vi "CodigoLabView 3.2.vi"() -> (11 "Releb 2":bool)   [LabVIEW 2025]
uses:
  <vilib>/Utility/NIReport.llb/Report Type.ctl
  <vilib>/Instr/_visa.llb/VISA Configure Serial Port (Instr).vi
  <vilib>/addons/_office/excel.llb/Excel Easy Table (str).vi
  <vilib>/Utility/NIReport.llb/NI_report.lvclass
  <vilib>/addons/_office/NI_ReportGenerationToolkit.lvlib
  <vilib>/Utility/NIReport.llb/NI_ReportGenerationCore.lvlib
  <vilib>/Utility/NIReport.llb/Excel/NI_Excel.lvclass
panel:
  out "Presionado":bool
  in  "RUTA DE REGISTRO":path
  out "Reloj Pot 4":dbl(knob) scale=0.0..100.0
  out "Reloj Pot 3":dbl(knob) scale=0.0..100.0
  out "Reloj Pot 2":dbl(knob) scale=0.0..100.0
  out "R ON 4":bool
  out "R ON 3":bool
  out "R ON 2":bool
  out "?":string
  out "R ON 1":bool
  out "TENSIÓN DE LÍNEA":dbl(knob) scale=100.0..300.0
  out "Reloj Pot 1":dbl(knob) scale=0.0..100.0
  in  "?":bool
  out "Releb 4":bool
  out "Relea 4":bool
  out "Rele 4":bool
  out "TOMACORRIENTE 4":bool
  out "Estado 4":string
  in  "Relé N°4":bool
  out "Potencia 4":string
  out "Releb 3":bool
  out "Relea 3":bool
  out "Rele 3":bool
  out "TOMACORRIENTE 3":bool
  out "Estado 3":string
  out "Potencia 3":string
  in  "Relé N°3":bool
  out "Relea 2":bool
  out "Rele 2":bool
  out "TOMACORRIENTE 2":bool
  out "Estado 2":string
  out "Potencia 2":string
  in  "Relé N°2":bool
  out "Releb 1":bool
  out "Relea 1":bool
  out "Rele 1":bool
  out "TOMACORRIENTE 1":bool
  out "Estado 1":string
  out "Potencia 1":string
  in  "Relé N°1":bool
  in  "PUERTO DE COMUNICACIÓN":refnum<visa-resource-name>
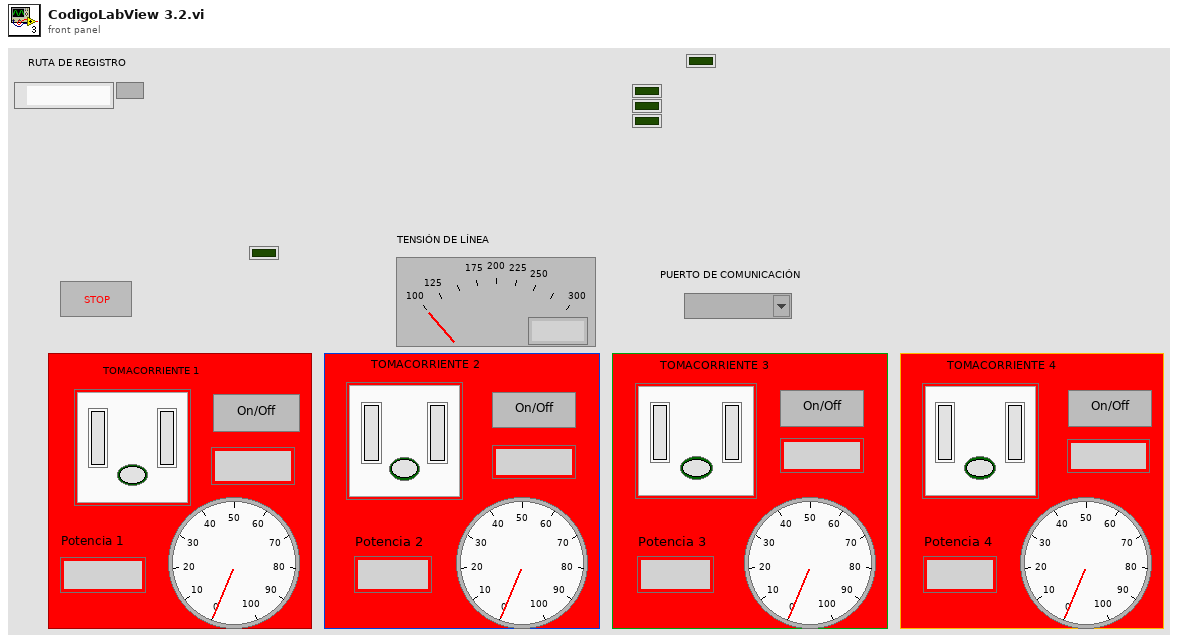
[diagram p1: front panel]
types:
  T1 = typedef "NI_ReportGenerationCore.lvlib/Report Type.ctl" = enum16{"HTML", "Word", "Excel"}
  T2 = cluster{"W1":string, "W2":string, "W3":string, "W4":string, "V":string}
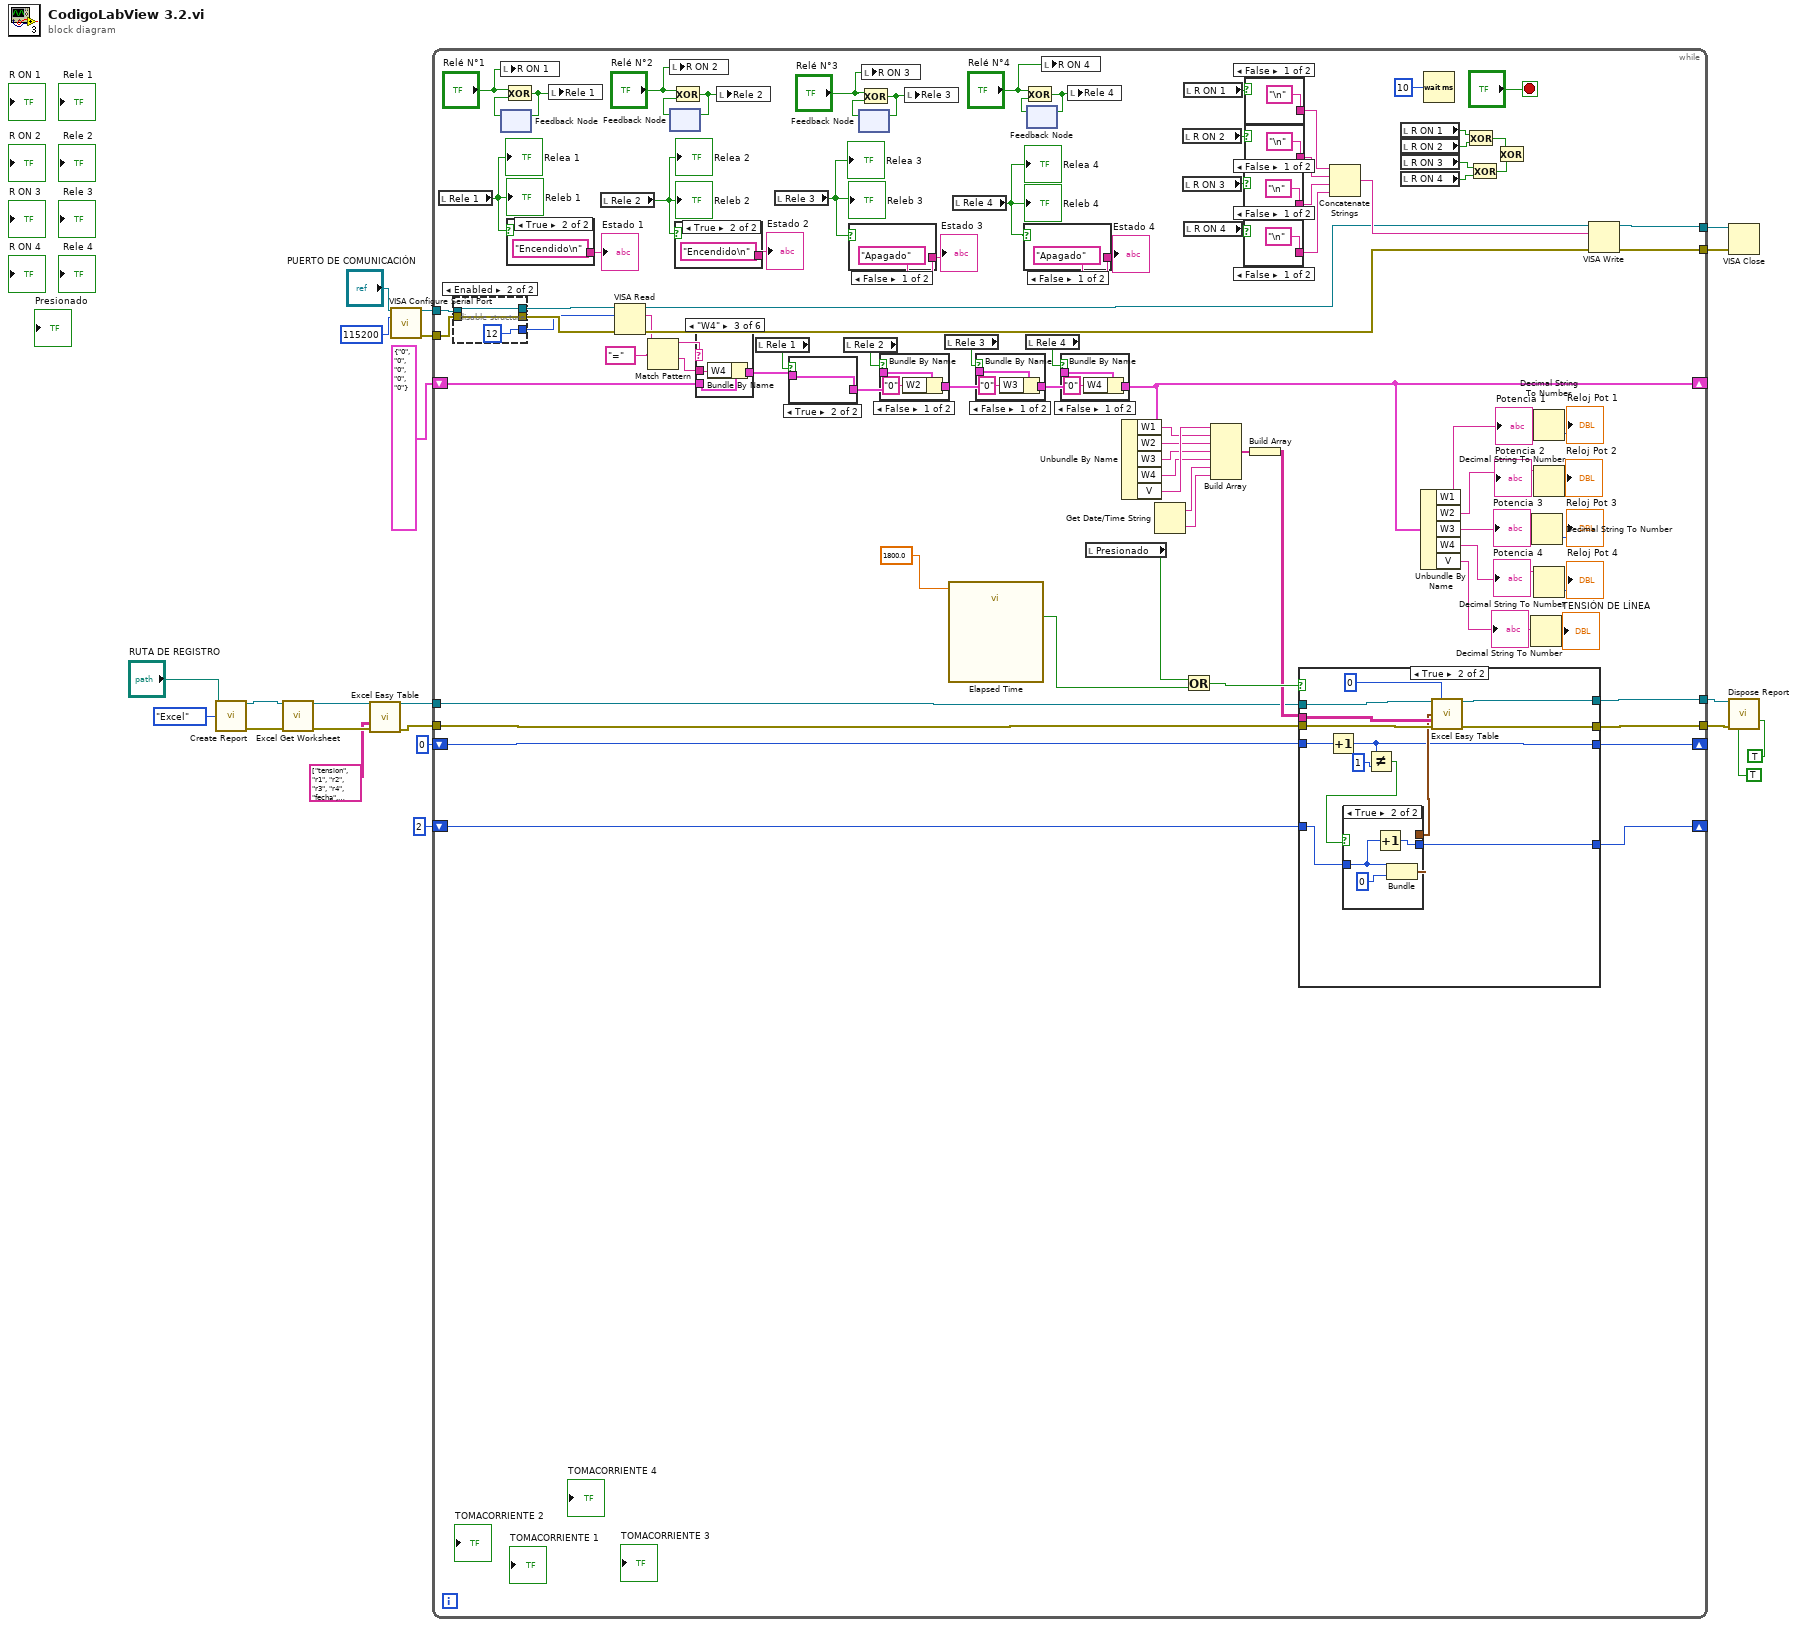
[diagram p0: block diagram]
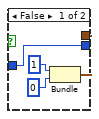
[diagram p3: hidden frame]
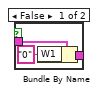
[diagram p5: hidden frame]
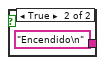
[diagram p8: hidden frame]
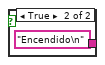
[diagram p9: hidden frame]
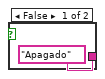
[diagram p10: hidden frame]
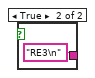
[diagram p11: hidden frame]
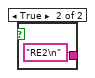
[diagram p12: hidden frame]
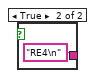
[diagram p13: hidden frame]
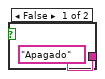
[diagram p14: hidden frame]
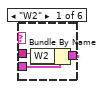
[diagram p15: hidden frame]
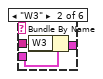
[diagram p16: hidden frame]
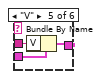
[diagram p18: hidden frame]
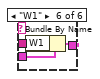
[diagram p19: hidden frame]
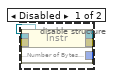
[diagram p20: hidden frame]
diagram:
  n1 = call <vilib>:"Create Report.vi"("report type"=Report_Type."Excel", "template (empty)"="RUTA DE REGISTRO") -> ("report out"=w11:refnum<class "NI_report.lvclass">, "error out"=w10:errorcluster)  [unwired: 12 in]
  n2 = call <vilib>:"Excel Get Worksheet.vi"("report in"=w11, "error in (no error)"=w10) -> ("report out"=w9:refnum<class "NI_report.lvclass">, "error out"=w8:errorcluster)  [unwired: 12 in]
  n3 = call-poly <vilib>:"Excel Easy Table.vi"("report in"=w9, "text data"=string[][] [["tension", "r1", "r2", "r3", "r4", "fecha", "hora"]], "error in (no error)"=w8) -> ("report out"=w4:refnum<class "NI_report.lvclass">, "error out"=w3:errorcluster)  [unwired: 8 in, 3 out]
  n4 = call-poly "VISA Configure Serial Port"("VISA resource name"="PUERTO DE COMUNICACIÓN", "baud rate (9600)"=u32 115200) -> ("VISA resource name out"=w22:refnum<visa-resource-name>, "error out"=w19:errorcluster)  [unwired: 12 in]
  n5 = while {
    tunnel: w22 -> [w113]
    tunnel: w19 -> [w112]
    shift-right: [w28] -> _
    shift-left: T2 {"W1"="0", "W2"="0", "W3"="0", "W4"="0", "V"="0"} -> [w108]
    tunnel: [w75] -> w17
    tunnel: [w74] -> w16
    shift-right: [w24] -> _
    shift-left: 0 -> [w23]
    shift-right: [w25] -> _
    shift-left: 2 -> [w38]
    tunnel: w4 -> [w37]
    tunnel: w3 -> [w36]
    tunnel: [w27] -> w2
    tunnel: [w26] -> w1
    stop <- "?" stop-if-true
    n6 = local read "Rele 1"() -> (w101:bool)
    "Releb 1" <- w101
    "Relea 1" <- w101
    n7 = disable-structure shown="Enabled" {
      disable-tunnel: w113 -> [w189 w192]
      disable-tunnel: w112 -> [w188 w191]
      disable-tunnel: [w187 w192] -> w73
      disable-tunnel: [w186 u32 12 ("Bytes at Port")] -> w71
      disable-tunnel: [w185 w191] -> w72
      frame Disabled {
        n8 = property class="Instr"(reference=w189, error in=w188) -> (reference out=w187:refnum<visa-resource-name>, error out=w185:errorcluster, "Serial Settings:Number of Bytes at Serial Port"=w186:u32)
      }
      frame Enabled {
      }
    }
    n9 = local write "R ON 1"("Relé N°1") -> ()
    n10 = feedback #1() -> (w105:bool)  [unwired: 1 in]
    n11 = Exclusive Or(1:w105, 2:"Relé N°1") -> (0:w102:bool)
    n12 = feedback-in #1(w102) -> ()
    n13 = case shown="True" w101 {
      tunnel: ["Apagado" "Encendido\n"] -> w104
      frame False {
      }
      frame True {
      }
    }
    "Estado 1" <- w104
    n14 = local write "Rele 1"(w102) -> ()
    n15 = local read "Rele 2"() -> (w93:bool)
    "Releb 2" <- w93
    "Relea 2" <- w93
    n16 = VISA Read(VISA resource name=w73, byte count=w71, error in (no error)=w72) -> (VISA resource name out=w70:refnum<visa-resource-name>, read buffer=w68:string, error out=w69:errorcluster)  [unwired: 1 out]
    n17 = Match Pattern(string=w68, regular expression="=") -> (before substring=w109:string, after substring=w77:string)  [unwired: 1 in, 2 out]
    n18 = local write "R ON 2"("Relé N°2") -> ()
    n19 = feedback #2() -> (w95:bool)  [unwired: 1 in]
    n20 = Exclusive Or(1:w95, 2:"Relé N°2") -> (0:w94:bool)
    n21 = feedback-in #2(w94) -> ()
    n22 = case shown="True" w93 {
      tunnel: ["Apagado" "Encendido\n"] -> w92
      frame False {
      }
      frame True {
      }
    }
    "Estado 2" <- w92
    n23 = case shown="\"W4\"" w109 {
      tunnel: w77 -> [w169 w172 w175 _ w179 w182]
      tunnel: w108 -> [w171 w174 w177 w178 w181 w184]
      tunnel: [w170 w173 w176 w178 w180 w183] -> w58
      frame "W2" {
        n24 = Bundle By Name(cluster=w171, "W2"=w169) -> (w170:T2)
      }
      frame "W3" {
        n25 = Bundle By Name(cluster=w174, "W3"=w172) -> (w173:T2)
      }
      frame "W4" {
        n26 = Bundle By Name(cluster=w177, "W4"=w175) -> (w176:T2)
      }
      frame "False", Default {
      }
      frame "V" {
        n27 = Bundle By Name(cluster=w181, "V"=w179) -> (w180:T2)
      }
      frame "W1" {
        n28 = Bundle By Name(cluster=w184, "W1"=w182) -> (w183:T2)
      }
    }
    n29 = local write "Rele 2"(w94) -> ()
    n30 = local read "Rele 1"() -> (w51:bool)
    n31 = local read "Rele 3"() -> (w88:bool)
    "Relea 3" <- w88
    "Releb 3" <- w88
    n32 = case shown="True" w51 {
      tunnel: w58 -> [w144 w146]
      tunnel: [w143 w146] -> w57
      frame False {
        n33 = Bundle By Name(cluster=w144, "W1"="0") -> (w143:T2)
      }
      frame True {
      }
    }
    n34 = local read "Rele 2"() -> (w52:bool)
    n35 = case shown="False" w88 {
      tunnel: ["Apagado" "Encendido\n"] -> w84
      frame False {
      }
      frame True {
      }
    }
    "Estado 3" <- w84
    n36 = feedback #3() -> (w90:bool)  [unwired: 1 in]
    n37 = Exclusive Or(1:w90, 2:"Relé N°3") -> (0:w89:bool)
    n38 = feedback-in #3(w89) -> ()
    n39 = local write "R ON 3"("Relé N°3") -> ()
    n40 = case shown="False" w52 {
      tunnel: w57 -> [w148 w150]
      tunnel: [w147 w150] -> w56
      frame False {
        n41 = Bundle By Name(cluster=w148, "W2"="0") -> (w147:T2)
      }
      frame True {
      }
    }
    n42 = local write "Rele 3"(w89) -> ()
    n43 = local read "Rele 3"() -> (w53:bool)
    n44 = call "Elapsed Time"("Time Target (s)"=1800.0) -> ("Time has Elapsed"=w49:bool)  [unwired: 11 in, 7 out]
    n45 = local read "Rele 4"() -> (w83:bool)
    "Relea 4" <- w83
    "Releb 4" <- w83
    n46 = case shown="False" w53 {
      tunnel: w56 -> [w140 w142]
      tunnel: [w139 w142] -> w55
      frame False {
        n47 = Bundle By Name(cluster=w140, "W3"="0") -> (w139:T2)
      }
      frame True {
      }
    }
    n48 = case shown="False" w83 {
      tunnel: ["Apagado" "Encendido\n"] -> w82
      frame False {
      }
      frame True {
      }
    }
    "Estado 4" <- w82
    n49 = local read "Rele 4"() -> (w54:bool)
    n50 = feedback #4() -> (w86:bool)  [unwired: 1 in]
    n51 = Exclusive Or(1:w86, 2:"Relé N°4") -> (0:w85:bool)
    n52 = feedback-in #4(w85) -> ()
    n53 = local write "R ON 4"("Relé N°4") -> ()
    n54 = case shown="False" w54 {
      tunnel: w55 -> [w152 w154]
      tunnel: [w151 w154] -> w28
      frame False {
        n55 = Bundle By Name(cluster=w152, "W4"="0") -> (w151:T2)
      }
      frame True {
      }
    }
    n56 = local write "Rele 4"(w85) -> ()
    n57 = local read "Presionado"() -> (w29:bool)
    n58 = Unbundle By Name(w28) -> ("W1"=w47:string, "W2"=w46:string, "W3"=w45:string, "W4"=w44:string, "V"=w48:string)
    n59 = Get Date/Time String() -> (date string=w42:string, time string=w43:string)  [unwired: 3 in]
    n60 = local read "R ON 2"() -> (w98:bool)
    n61 = local read "R ON 3"() -> (w97:bool)
    n62 = local read "R ON 1"() -> (w100:bool)
    n63 = local read "R ON 4"() -> (w99:bool)
    n64 = Or(x=w29, y=w49) -> (x .or. y?=w50:bool)
    n65 = Build Array(w48, w47, w46, w45, w44, w42, w43) -> (w40:string[])
    n66 = case shown="False" w97 {
      tunnel: ["\n" "RE3\n"] -> w79
      frame False {
      }
      frame True {
      }
    }
    n67 = case shown="False" w99 {
      tunnel: ["\n" "RE4\n"] -> w80
      frame False {
      }
      frame True {
      }
    }
    n68 = case shown="False" w100 {
      tunnel: ["\n" "RE1\n"] -> w107
      frame False {
      }
      frame True {
      }
    }
    n69 = case shown="False" w98 {
      tunnel: ["\n" "RE2\n"] -> w81
      frame False {
      }
      frame True {
      }
    }
    n70 = Build Array(w40) -> (w41:string[][])
    n71 = case shown="True" w50 {
      tunnel: w41 -> [_ w130]
      tunnel: w36 -> [w117 w129]
      tunnel: [w116 w128] -> w27
      tunnel: [w117 w127] -> w26
      tunnel: w37 -> [w116 w126]
      tunnel: w38 -> [w115 w123]
      tunnel: [w115 w122] -> w25
      tunnel: w23 -> [w114 w121]
      tunnel: [w114 w118] -> w24
      frame False {
      }
      frame True {
        n72 = Increment(x=w121) -> (x+1=w118:i32)
        n73 = Not Equal?(x=w118, y=1) -> (x != y?=w119:bool)
        n74 = case shown="True" w119 {
          tunnel: [w132 w138] -> w125
          tunnel: w123 -> [w131 w136]
          tunnel: [w131 w135] -> w122
          frame False {
            n75 = Bundle(1, 0) -> (w132:cluster{i32, i32})  [unwired: 1 in]
          }
          frame True {
            n76 = Increment(x=w136) -> (x+1=w135:i32)
            n77 = Bundle(w136, 0) -> (w138:cluster{i32, i32})  [unwired: 1 in]
          }
        }
        n78 = call-poly <vilib>:"Excel Easy Table.vi"("report in"=w126, "iteration"=0, "start (0, 0)"=w125, "text data"=w130, "error in (no error)"=w129) -> ("report out"=w128:refnum<class "NI_report.lvclass">, "error out"=w127:errorcluster)  [unwired: 6 in, 3 out]
      }
    }
    n79 = Concatenate Strings(w107, w81, w79, w80) -> (w76:string)
    n80 = local read "R ON 1"() -> (w35:bool)
    n81 = local read "R ON 2"() -> (w34:bool)
    n82 = local read "R ON 3"() -> (w32:bool)
    n83 = local read "R ON 4"() -> (w33:bool)
    n84 = Unbundle By Name(w28) -> ("W1"=w67:string, "W2"=w62:string, "W3"=w61:string, "W4"=w60:string, "V"=w59:string)
    "Potencia 1" <- w67
    "?" <- w59
    "Potencia 2" <- w62
    "Potencia 3" <- w61
    "Potencia 4" <- w60
    n85 = Wait (ms)(milliseconds to wait=u32 10) -> ()  [unwired: 1 out]
    n86 = Exclusive Or(1:w34, 2:w35) -> (0:w30:bool)
    n87 = Exclusive Or(1:w33, 2:w32) -> (0:w31:bool)
    n88 = Exclusive Or(1:w31, 2:w30) -> ()  [unwired: 1 out]
    n89 = Decimal String To Number(string=w59) -> (number=→"TENSIÓN DE LÍNEA":i32)  [unwired: 2 in, 1 out]
    n90 = Decimal String To Number(string=w61) -> (number=→"Reloj Pot 3":i32)  [unwired: 2 in, 1 out]
    n91 = Decimal String To Number(string=w67) -> (number=→"Reloj Pot 1":i32)  [unwired: 2 in, 1 out]
    n92 = Decimal String To Number(string=w62) -> (number=→"Reloj Pot 2":i32)  [unwired: 2 in, 1 out]
    n93 = Decimal String To Number(string=w60) -> (number=→"Reloj Pot 4":i32)  [unwired: 2 in, 1 out]
    n94 = VISA Write(VISA resource name=w70, write buffer=w76, error in (no error)=w69) -> (VISA resource name out=w75:refnum<visa-resource-name>, error out=w74:errorcluster)  [unwired: 1 out]
  }
  n95 = VISA Close(VISA resource name=w17, error in (no error)=w16) -> ()  [unwired: 1 out]
  n96 = call-dynamic "Dispose Report.vi"("report in"=w2, "save changes? (F)"=TRUE, "error in (no error)"=w1, "close report? (T)"=TRUE) -> ()  [unwired: 11 in, 1 out]
